vi "Ejercicio_17_PWM.vi"() -> ()   [LabVIEW 2020]
panel:
  in  "Amplitude":dbl=1.0
  out "Waveform Graph":dynamicdata(graph)
  in  "Periodo":dbl=10.1 caption="Frequency"
  in  "Duty Cycle (%)":dbl=50.0
  in  "STOP":bool
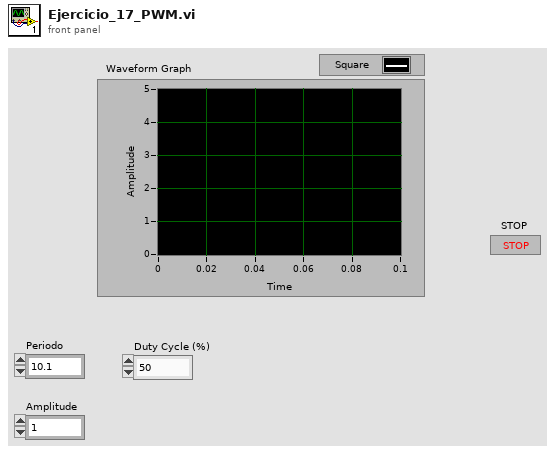
[diagram p1: front panel]
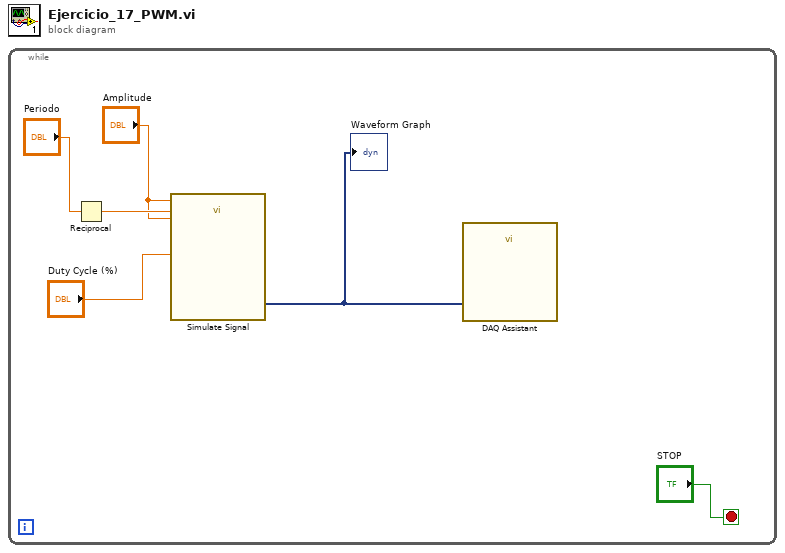
[diagram p0: block diagram]
diagram:
  n1 = while {
    stop <- "STOP" stop-if-true
    n2 = Reciprocal(x="Periodo") -> (1/x=w3:dbl)
    n3 = call "Simulate Signal"("Offset"="Amplitude", "Duty Cycle (%)"="Duty Cycle (%)", "Frequency"=w3, "Amplitude"="Amplitude") -> ("Square"=w2:dynamicdata)  [unwired: 10 in, 1 out]
    "Waveform Graph" <- w2
    n4 = call "DAQ Assistant"("data"=w2) -> ()  [unwired: 17 in, 2 out]
  }
